vi "Ring Value Update.vi"(7 "Ring in":refnum<vi>, 8 "error in (no error)":errorcluster, 11 "SlaveID":i32) -> (0 "error out":errorcluster)   [LabVIEW 2020, in "Master.lvlib"]
uses:
  Master.lvlib
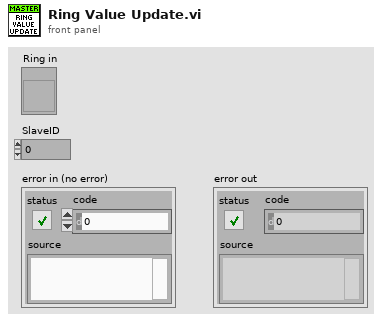
[diagram p1: front panel]
types:
  T1 = typedef "LVStringsAndValuesArrayTypeDef_I32.ctl" = cluster{"String":string, "Value":i32}[]
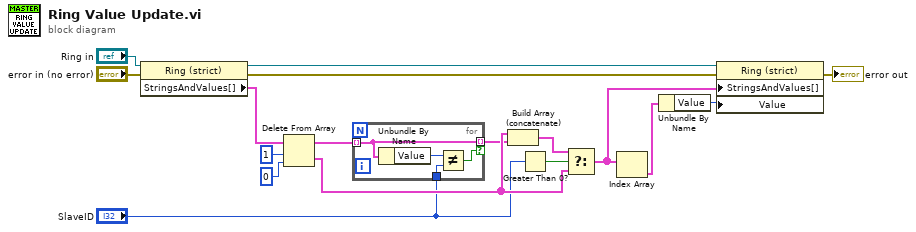
[diagram p0: block diagram]
diagram:
  n1 = property on="Property Node" class="Ring (strict)"(reference="Ring in", error in="error in (no error)") -> (reference out=w1:refnum<vi>, error out=w9:errorcluster, "StringsAndValues[]"=w12:T1)
  n2 = Delete From Array(array=w12, length=1, index=0) -> (deleted portion=w17:T1, array with subset deleted=w14:T1)
  n3 = for {
    tunnel: w14 -> [w19] mode=indexing
    tunnel: "SlaveID" -> [w20]
    tunnel: [w19] -> w11 mode=indexing if=w18
    n4 = Unbundle By Name(w19) -> ("Value"=w21:i32)
    n5 = Not Equal?(x=w21, y=w20) -> (x != y?=w18:bool)
  }
  n6 = Build Array (concatenate)(w17, w11) -> (w16:T1)
  n7 = Greater Than 0?(x="SlaveID") -> (x > 0?=w5:bool)
  n8 = Select(t=w16, s=w5, f=w17) -> (s? t:f=w3:T1)
  n9 = Index Array(array=w3) -> (element=w4:cluster{"String":string, "Value":i32})  [unwired: 1 in]
  n10 = Unbundle By Name(w4) -> ("Value"=w2:i32)
  n11 = property on="Property Node" class="Ring (strict)"(reference=w1, error in=w9, "StringsAndValues[]"=w3, "Value"=w2) -> (error out=→"error out":errorcluster)  [unwired: 1 out]
